vi "Functional Test Aging.vi"(8 "connection information":path, 9 "error in":errorcluster, 10 "Arduino":refnum<visa-resource-name>, 11 "System Number":string) -> (1 "error out":errorcluster, 2 "Arduino":refnum<visa-resource-name>, 3 "Functional Test Data":string)   [LabVIEW 2024]
uses:
  <vilib>/addons/database/Connection.llb/DB Tools Open Connec (Path).vi
  <vilib>/addons/database/_DB Variant To Data/Database Variant To Data.xnode
  <vilib>/addons/database/NI_Database_API.lvlib
panel:
  out "Functional Test Data Rack 1":string
  out "Functional Test Data Rack 2":string
  out "Upper Position":i32
  out "Upper Rack":dbl
  out "Lower Rack":dbl
  out "Lower Position":i32
  out "OscVoltage":string
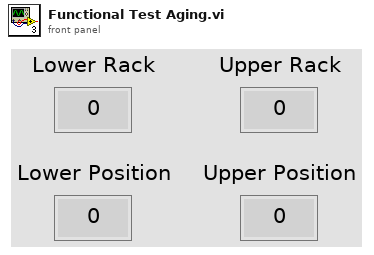
[diagram p1: front panel]
types:
  T1 = typedef "NI_Database_API.lvlib/Conn ObjectReference.ctl" = refnum<k1>
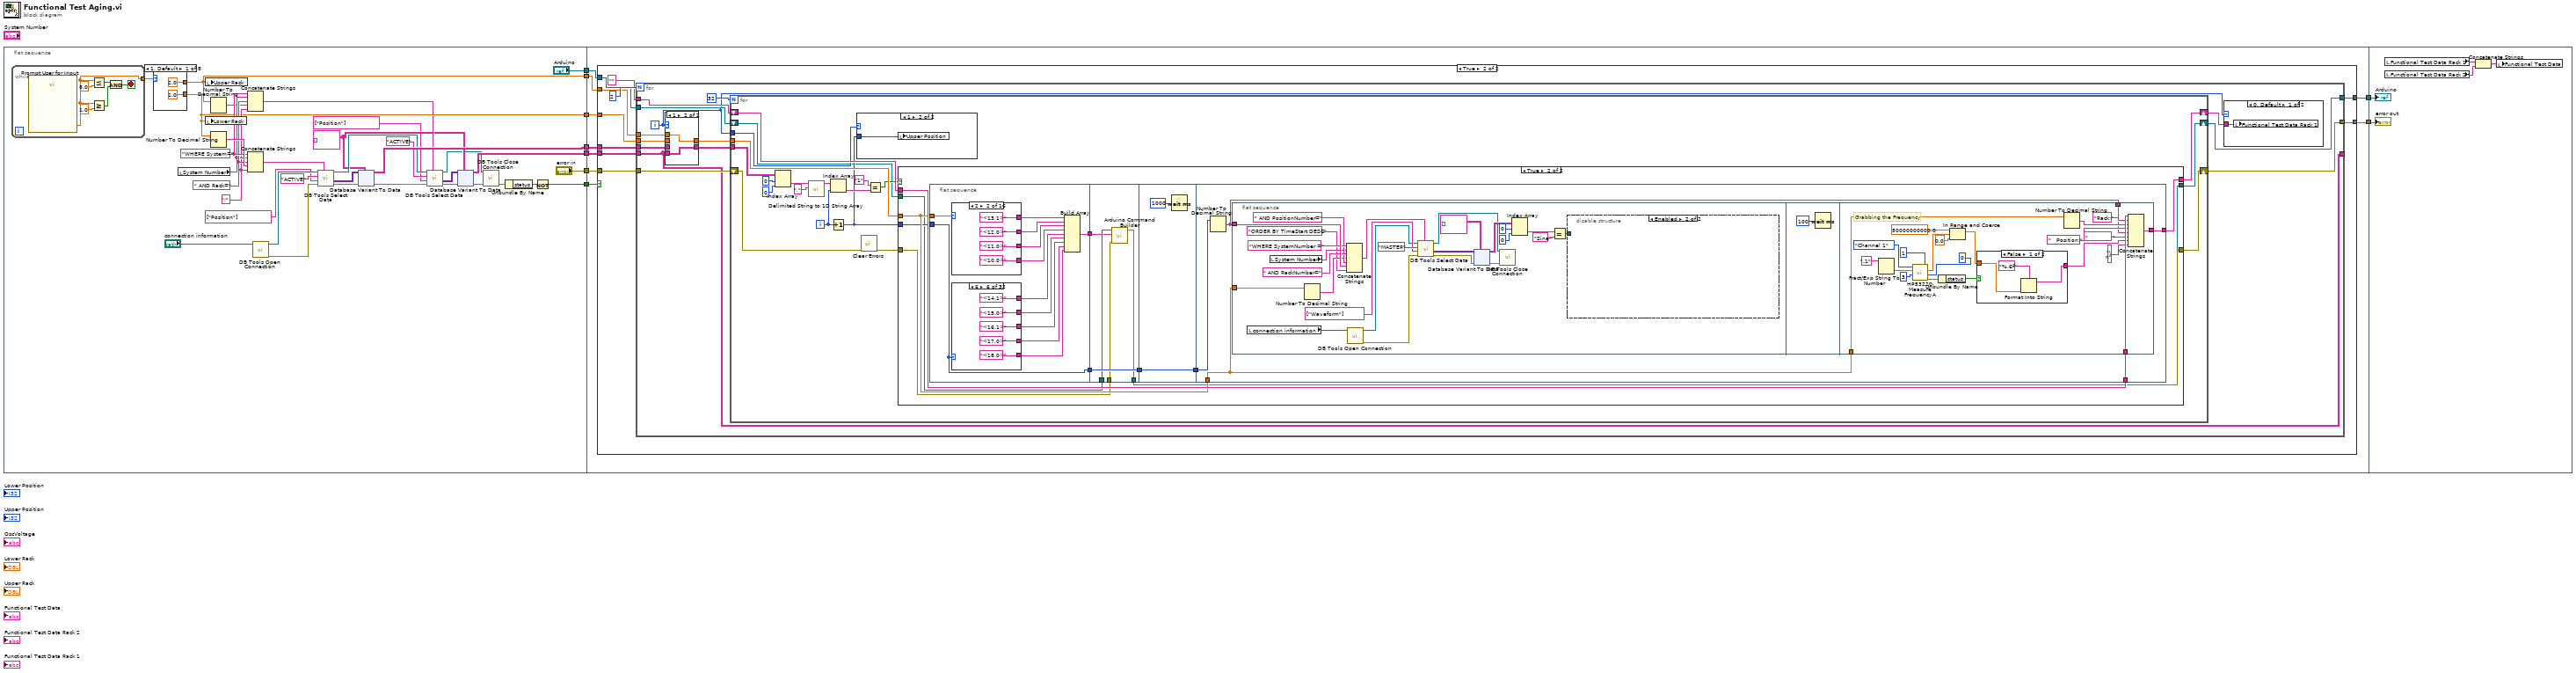
[diagram p0: block diagram]
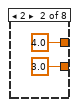
[diagram p2: hidden frame]
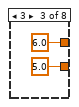
[diagram p3: hidden frame]
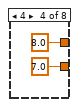
[diagram p4: hidden frame]
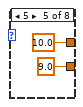
[diagram p5: hidden frame]
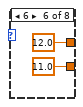
[diagram p6: hidden frame]
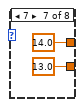
[diagram p7: hidden frame]
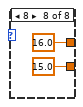
[diagram p8: hidden frame]
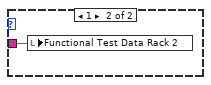
[diagram p10: hidden frame]
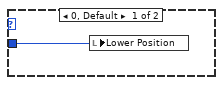
[diagram p12: hidden frame]
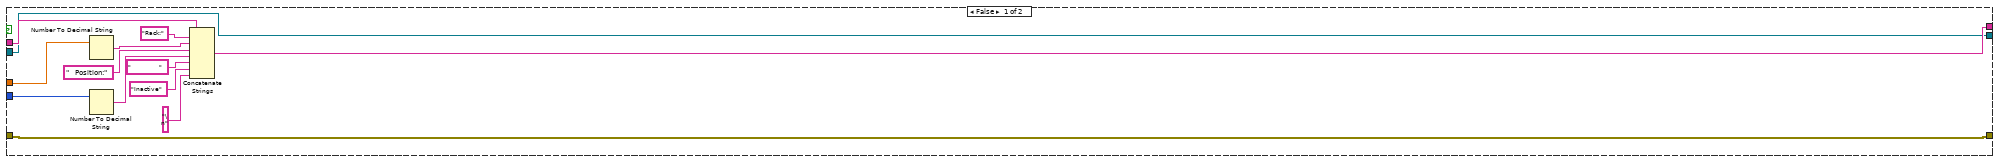
[diagram p13: hidden frame]
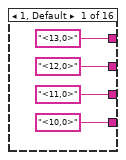
[diagram p14: hidden frame]
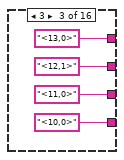
[diagram p15: hidden frame]
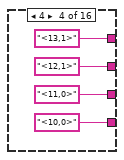
[diagram p16: hidden frame]
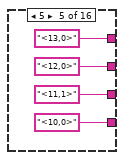
[diagram p17: hidden frame]
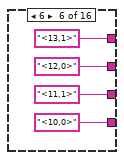
[diagram p18: hidden frame]
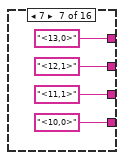
[diagram p19: hidden frame]
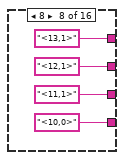
[diagram p20: hidden frame]
diagram:
  n1 = flat-sequence {
    tunnel: [w24] -> w9
    tunnel: ["Arduino"] -> w8
    tunnel: ["error in"] -> w7
    tunnel: [w16] -> w6
    tunnel: [w33] -> w5
    tunnel: [w35] -> w4
    tunnel: [w31] -> w1
    tunnel: w9 -> [w160]
    tunnel: w8 -> [w156]
    tunnel: w7 -> [w155]
    tunnel: w6 -> [w159]
    tunnel: w5 -> [w158]
    tunnel: w4 -> [w157]
    tunnel: [w162] -> w3
    tunnel: [w161] -> w2
    tunnel: w1 -> [w154]
    tunnel: w3 -> [w603]
    tunnel: w2 -> [w604]
    frame #0 {
      w15 = string[][] [] ("table")
      w39 = " AND Rack="
      w37 = ";" ("string")
      w40 = "WHERE System=" ("SQL Query")
      n2 = while {
        tunnel: [w153] -> w36
        stop <- w150 stop-if-true
        n3 = call "Prompt User for Input"() -> ("Shelf Number"=w153:dbl)  [unwired: 17 in, 2 out]
        n4 = Less Or Equal?(x=w153, y=8.0) -> (x <= y?=w149:bool)
        n5 = Greater Or Equal?(x=w153, y=1.0) -> (x >= y?=w148:bool)
        n6 = And(x=w149, y=w148) -> (x .and. y?=w150:bool)
      }
      n7 = case shown="1, Default" w36 {
        tunnel: [1.0 ("y") 3.0 ("y") 5.0 ("y") 7.0 ("y") 9.0 ("y") 11.0 ("y") 13.0 ("y") 15.0 ("y")] -> w35
        tunnel: [2.0 ("y") 4.0 ("y") 6.0 ("y") 8.0 ("y") 10.0 ("y") 12.0 ("y") 14.0 ("y") 16.0 ("y")] -> w33
        frame 1, Default {
        }
        frame 2 {
        }
        frame 3 {
        }
        frame 4 {
        }
        frame 5 {
        }
        frame 6 {
        }
        frame 7 {
        }
        frame 8 {
        }
      }
      n8 = local read "System Number"() -> (w38:string)
      n9 = local write "Upper Rack"(w33) -> ()
      n10 = local write "Lower Rack"(w35) -> ()
      n11 = Number To Decimal String(number=w33) -> (decimal integer string=w34:string)  [unwired: 1 in]
      n12 = Number To Decimal String(number=w35) -> (decimal integer string=w43:string)  [unwired: 1 in]
      n13 = Concatenate Strings(w40, w38, w39, w34, w37) -> (w21:string)
      n14 = Concatenate Strings(w40, w38, w39, w43, w37) -> (w25:string)
      n15 = call-poly <vilib>:"DB Tools Open Connection.vi"("connection information"="connection information") -> ("error out"=w28:errorcluster, "connection reference"=w29:T1)  [unwired: 7 in]
      n16 = call <vilib>:"DB Tools Select Data.vi"("condition"=w25, "error in (no error)"=w28, "columns"=string[] ["Position"], "table"="ACTIVE", "connection reference"=w29) -> ("error out"=w20:errorcluster, "data"=w26:variant[][], "connection reference out"=w23:T1)  [unwired: 1 in]
      n17 = xnode "Database Variant To Data"("database variant"=w26, "error in (no error)"=w20, "type"=w15) -> ("data"=w24:string[][], "error out"=w19:errorcluster)
      n18 = call <vilib>:"DB Tools Select Data.vi"("condition"=w21, "error in (no error)"=w19, "columns"=string[] ["Position"], "table"="ACTIVE", "connection reference"=w23) -> ("error out"=w18:errorcluster, "data"=w17:variant[][], "connection reference out"=w12:T1)  [unwired: 1 in]
      n19 = xnode "Database Variant To Data"("database variant"=w17, "error in (no error)"=w18, "type"=w15) -> ("data"=w16:string[][], "error out"=w11:errorcluster)
      n20 = call <vilib>:"DB Tools Close Connection.vi"("error in (no error)"=w11, "connection reference"=w12) -> ("error out"=w10:errorcluster)  [unwired: 5 in]
      n21 = Unbundle By Name(w10) -> ("status"=w32:bool)
      n22 = Not(x=w32) -> (.not. x?=w31:bool)
    }
    frame #1 {
      n23 = case shown="True" w154 {
        tunnel: [w163 w172] -> w162
        tunnel: [w164 w171] -> w161
        tunnel: w160 -> [_ w170]
        tunnel: w159 -> [_ w169]
        tunnel: w158 -> [_ w168]
        tunnel: w157 -> [_ w167]
        tunnel: w156 -> [w163 w166]
        tunnel: w155 -> [w164 w165]
        frame False {
        }
        frame True {
          n24 = for {
            N: 2 -> [_]
            tunnel: "" -> [w188]
            tunnel: [w187] -> w172
            tunnel: [w186] -> w171
            tunnel: w170 -> [w182]
            tunnel: w165 -> [w184]
            tunnel: w166 -> [w183]
            tunnel: [w177] -> _
            tunnel: w169 -> [w177]
            tunnel: w168 -> [w176]
            tunnel: w167 -> [w175]
            i -> [w178]
            n25 = case shown="1" w178 {
              tunnel: w182 -> [w192 _]
              tunnel: w177 -> [_ w194]
              tunnel: [w192 w194] -> w181
              tunnel: w176 -> [_ w193]
              tunnel: w175 -> [w191 _]
              tunnel: [w191 w193] -> w180
              frame 0, Default {
              }
              frame 1 {
              }
            }
            n26 = for {
              N: 32 -> [_]
              shift-right: [w203] -> w179
              shift-left: w188 -> [w204]
              tunnel: w180 -> [w205]
              tunnel: w181 -> [w209]
              shift-right: [w201] -> w187
              shift-left: w183 -> [w196]
              shift-right: [w202] -> w186
              shift-left: w184 -> [w214]
              tunnel: w178 -> [w197]
              i -> [w199]
              n27 = Index Array(array=w209, index (row)=0 ("disabled index (row)"), index (col)=0 ("disabled index (col)")) -> (element=w211:string)
              n28 = call <vilib>:"Delimited String to 1D String Array.vi"("delimiter"=",", "delimited string"=w211) -> ("string array"=w212:string[])  [unwired: 9 in]
              n29 = Index Array(array=w212, index=w199) -> (element=w213:string)
              n30 = Increment(x=w199) -> (x+1=w198:i32)
              n31 = case shown="1" w197 {
                tunnel: w198 -> [w215 w216]
                frame 0, Default {
                  n32 = local write "Lower Position"(w215) -> ()
                }
                frame 1 {
                  n33 = local write "Upper Position"(w216) -> ()
                }
              }
              n34 = call <vilib>:"Clear Errors.vi"("error in (no error)"=w214) -> ("error out"=w195:errorcluster)  [unwired: 5 in, 1 out]
              n35 = Equal?(x="1", y=w213) -> (x = y?=w200:bool)
              n36 = case shown="True" w200 {
                tunnel: w198 -> [w217 w238]
                tunnel: w205 -> [w220 w240]
                tunnel: w204 -> [w221 w241]
                tunnel: w196 -> [w218 w235]
                tunnel: w195 -> [w219 w236]
                tunnel: [w223 w239] -> w203
                tunnel: [w219 w234] -> w202
                tunnel: [w218 w233] -> w201
                frame False {
                  n37 = Number To Decimal String(number=w220) -> (decimal integer string=w228:string)  [unwired: 1 in]
                  n38 = Number To Decimal String(number=w217) -> (decimal integer string=w222:string)  [unwired: 1 in]
                  n39 = Concatenate Strings(w221, "Rack:" ("string"), w228, "   Position:" ("string"), w222, "              " ("string"), "Inactive" ("string"), "\n" ("string")) -> (w223:string)
                }
                frame True {
                  n40 = flat-sequence {
                    tunnel: w238 -> [w243]
                    tunnel: w240 -> [w244]
                    tunnel: [w243] -> w237
                    tunnel: [w242] -> w232
                    tunnel: [w483] -> w231
                    tunnel: w237 -> [w483]
                    tunnel: w236 -> [w482]
                    tunnel: w235 -> [w481]
                    tunnel: [w480] -> w234
                    tunnel: [w479] -> w233
                    tunnel: w232 -> [w478]
                    tunnel: w231 -> [w485]
                    tunnel: [w485] -> w230
                    tunnel: w241 -> [w490]
                    tunnel: w240 -> [w489]
                    tunnel: [w488] -> w239
                    tunnel: w230 -> [w486]
                    frame #0 {
                      n41 = case shown="2" w244 {
                        tunnel: ["<10,0>" ("string") "<10,0>" ("string") "<10,0>" ("string") "<10,0>" ("string") "<10,0>" ("string") "<10,0>" ("string") "<10,0>" ("string") "<10,0>" ("string") "<10,1>" ("string") "<10,1>" ("string") "<10,1>" ("string") "<10,1>" ("string") "<10,1>" ("string") "<10,1>" ("string") "<10,1>" ("string") "<10,1>" ("string")] -> w251
                        tunnel: ["<12,0>" ("string") "<12,0>" ("string") "<12,1>" ("string") "<12,1>" ("string") "<12,0>" ("string") "<12,0>" ("string") "<12,1>" ("string") "<12,1>" ("string") "<12,0>" ("string") "<12,0>" ("string") "<12,1>" ("string") "<12,1>" ("string") "<12,0>" ("string") "<12,0>" ("string") "<12,1>" ("string") "<12,1>" ("string")] -> w252
                        tunnel: ["<11,0>" ("string") "<11,0>" ("string") "<11,0>" ("string") "<11,0>" ("string") "<11,1>" ("string") "<11,1>" ("string") "<11,1>" ("string") "<11,1>" ("string") "<11,0>" ("string") "<11,0>" ("string") "<11,0>" ("string") "<11,0>" ("string") "<11,1>" ("string") "<11,1>" ("string") "<11,1>" ("string") "<11,1>" ("string")] -> w253
                        tunnel: ["<13,0>" ("string") "<13,1>" ("string") "<13,0>" ("string") "<13,1>" ("string") "<13,0>" ("string") "<13,1>" ("string") "<13,0>" ("string") "<13,1>" ("string") "<13,0>" ("string") "<13,1>" ("string") "<13,0>" ("string") "<13,1>" ("string") "<13,0>" ("string") "<13,1>" ("string") "<13,0>" ("string") "<13,1>" ("string")] -> w250
                        frame 1, Default {
                        }
                        frame 2 {
                        }
                        frame 3 {
                        }
                        frame 4 {
                        }
                        frame 5 {
                        }
                        frame 6 {
                        }
                        frame 7 {
                        }
                        frame 8 {
                        }
                        frame 9 {
                        }
                        frame 10 {
                        }
                        frame 11 {
                        }
                        frame 12 {
                        }
                        frame 13 {
                        }
                        frame 14 {
                        }
                        frame 15 {
                        }
                        frame 16 {
                        }
                      }
                      n42 = case shown="6" w243 {
                        tunnel: ["<14,0>" ("string") "<14,1>" ("string") "<14,0>" ("string") "<14,1>" ("string") "<14,0>" ("string") "<14,1>" ("string") "<14,0>" ("string") "<14,1>" ("string") "<14,0>" ("string") "<14,1>" ("string") "<14,0>" ("string") "<14,1>" ("string") "<14,0>" ("string") "<14,1>" ("string") "<14,0>" ("string") "<14,1>" ("string") "<14,0>" ("string") "<14,1>" ("string") "<14,0>" ("string") "<14,1>" ("string") "<14,0>" ("string") "<14,1>" ("string") "<14,0>" ("string") "<14,1>" ("string") "<14,0>" ("string") "<14,1>" ("string") "<14,0>" ("string") "<14,1>" ("string") "<14,0>" ("string") "<14,1>" ("string") "<14,0>" ("string") "<14,1>" ("string")] -> w249
                        tunnel: ["<16,0>" ("string") "<16,0>" ("string") "<16,0>" ("string") "<16,0>" ("string") "<16,1>" ("string") "<16,1>" ("string") "<16,1>" ("string") "<16,1>" ("string") "<16,0>" ("string") "<16,0>" ("string") "<16,0>" ("string") "<16,0>" ("string") "<16,1>" ("string") "<16,1>" ("string") "<16,1>" ("string") "<16,1>" ("string") "<16,0>" ("string") "<16,0>" ("string") "<16,0>" ("string") "<16,0>" ("string") "<16,1>" ("string") "<16,1>" ("string") "<16,1>" ("string") "<16,1>" ("string") "<16,0>" ("string") "<16,0>" ("string") "<16,0>" ("string") "<16,0>" ("string") "<16,1>" ("string") "<16,1>" ("string") "<16,1>" ("string") "<16,1>" ("string")] -> w247
                        tunnel: ["<18,0>" ("string") "<18,0>" ("string") "<18,0>" ("string") "<18,0>" ("string") "<18,0>" ("string") "<18,0>" ("string") "<18,0>" ("string") "<18,0>" ("string") "<18,0>" ("string") "<18,0>" ("string") "<18,0>" ("string") "<18,0>" ("string") "<18,0>" ("string") "<18,0>" ("string") "<18,0>" ("string") "<18,0>" ("string") "<18,1>" ("string") "<18,1>" ("string") "<18,1>" ("string") "<18,1>" ("string") "<18,1>" ("string") "<18,1>" ("string") "<18,1>" ("string") "<18,1>" ("string") "<18,1>" ("string") "<18,1>" ("string") "<18,1>" ("string") "<18,1>" ("string") "<18,1>" ("string") "<18,1>" ("string") "<18,1>" ("string") "<18,1>" ("string")] -> w245
                        tunnel: ["<15,0>" ("string") "<15,0>" ("string") "<15,1>" ("string") "<15,1>" ("string") "<15,0>" ("string") "<15,0>" ("string") "<15,1>" ("string") "<15,1>" ("string") "<15,0>" ("string") "<15,0>" ("string") "<15,1>" ("string") "<15,1>" ("string") "<15,0>" ("string") "<15,0>" ("string") "<15,1>" ("string") "<15,1>" ("string") "<15,0>" ("string") "<15,0>" ("string") "<15,1>" ("string") "<15,1>" ("string") "<15,0>" ("string") "<15,0>" ("string") "<15,1>" ("string") "<15,1>" ("string") "<15,0>" ("string") "<15,0>" ("string") "<15,1>" ("string") "<15,1>" ("string") "<15,0>" ("string") "<15,0>" ("string") "<15,1>" ("string") "<15,1>" ("string")] -> w248
                        tunnel: ["<17,0>" ("string") "<17,0>" ("string") "<17,0>" ("string") "<17,0>" ("string") "<17,0>" ("string") "<17,0>" ("string") "<17,0>" ("string") "<17,0>" ("string") "<17,1>" ("string") "<17,1>" ("string") "<17,1>" ("string") "<17,1>" ("string") "<17,1>" ("string") "<17,1>" ("string") "<17,1>" ("string") "<17,1>" ("string") "<17,0>" ("string") "<17,0>" ("string") "<17,0>" ("string") "<17,0>" ("string") "<17,0>" ("string") "<17,0>" ("string") "<17,0>" ("string") "<17,0>" ("string") "<17,1>" ("string") "<17,1>" ("string") "<17,1>" ("string") "<17,1>" ("string") "<17,1>" ("string") "<17,1>" ("string") "<17,1>" ("string") "<17,1>" ("string")] -> w246
                        frame 1, Default {
                        }
                        frame 2 {
                        }
                        frame 3 {
                        }
                        frame 4 {
                        }
                        frame 5 {
                        }
                        frame 6 {
                        }
                        frame 7 {
                        }
                        frame 8 {
                        }
                        frame 9 {
                        }
                        frame 10 {
                        }
                        frame 11 {
                        }
                        frame 12 {
                        }
                        frame 13 {
                        }
                        frame 14 {
                        }
                        frame 15 {
                        }
                        frame 16 {
                        }
                        frame 17 {
                        }
                        frame 18 {
                        }
                        frame 19 {
                        }
                        frame 20 {
                        }
                        frame 21 {
                        }
                        frame 22 {
                        }
                        frame 23 {
                        }
                        frame 24 {
                        }
                        frame 25 {
                        }
                        frame 26 {
                        }
                        frame 27 {
                        }
                        frame 28 {
                        }
                        frame 29 {
                        }
                        frame 30 {
                        }
                        frame 31 {
                        }
                        frame 32 {
                        }
                      }
                      n43 = Build Array(w250, w252, w253, w251, w249, w248, w247, w246, w245) -> (w242:string[])
                    }
                    frame #1 {
                      n44 = call "Arduino Command Builder.vi"("error in"=w482, "Commands"=w478, "Arduino in"=w481) -> ("error out"=w480:errorcluster, "Arduino out"=w479:refnum<visa-resource-name>)  [unwired: 7 in]
                    }
                    frame #2 {
                      n45 = Wait (ms)(milliseconds to wait=u32 1000) -> ()  [unwired: 1 out]
                    }
                    frame #3 {
                      n46 = Number To Decimal String(number=w486) -> (decimal integer string=w487:string)  [unwired: 1 in]
                      n47 = flat-sequence {
                        tunnel: w489 -> [w515]
                        tunnel: w487 -> [w514]
                        tunnel: [w595] -> w488
                        tunnel: w489 -> [w576]
                        tunnel: w490 -> [w593]
                        tunnel: w487 -> [w577]
                        frame #0 {
                          n48 = local read "connection information"() -> (w491:path)
                          n49 = local read "System Number"() -> (w509:string)
                          n50 = Number To Decimal String(number=w515) -> (decimal integer string=w508:string)  [unwired: 1 in]
                          n51 = Concatenate Strings("WHERE SystemNumber =" ("SQL Query"), w509, " AND RackNumber=" ("string"), w508, " AND PositionNumber=" ("string"), w514, "ORDER BY TimeStart DESC" ("string")) -> (w499:string)
                          n52 = call-poly <vilib>:"DB Tools Open Connection.vi"("connection information"=w491) -> ("error out"=w494:errorcluster, "connection reference"=w495:T1)  [unwired: 7 in]
                          n53 = call <vilib>:"DB Tools Select Data.vi"("condition"=w499, "error in (no error)"=w494, "columns"=string[] ["Waveform"], "table"="MASTER", "connection reference"=w495) -> ("error out"=w500:errorcluster, "data"=w501:variant[][], "connection reference out"=w493:T1)  [unwired: 1 in]
                          n54 = xnode "Database Variant To Data"("database variant"=w501, "error in (no error)"=w500, "type"=string[][] [] ("table")) -> ("data"=w498:string[][], "error out"=w492:errorcluster)
                          n55 = call <vilib>:"DB Tools Close Connection.vi"("error in (no error)"=w492, "connection reference"=w493) -> ()  [unwired: 5 in, 1 out]
                          n56 = Index Array(array=w498, index (row)=0, index (col)=0) -> (element=w504:string)
                          n57 = Equal?(x=w504, y="Sine") -> (x = y?=w513:bool)
                          n58 = disable-structure shown="Enabled" {
                            disable-tunnel: w513 -> [w516 _]
                            frame Disabled {
                              n59 = case shown="False" w516 {
                                frame False {
                                n60 = flat-sequence {
                                frame #0 {
                                n61 = Send(0:0 ("bus"), 2:i16 3 ("address"), 5:"INP1:COUP DC " ("data string")) -> ()  [unwired: 2 in, 3 out]
                                }
                                frame #1 {
                                n62 = Send(0:0 ("bus"), 2:i16 3 ("address"), 5:"INP1:IMP MAX" ("data string")) -> ()  [unwired: 2 in, 3 out]
                                }
                                }
                                }
                                frame True {
                                n63 = flat-sequence {
                                frame #0 {
                                n64 = Send(0:0 ("bus"), 2:i16 3 ("address"), 5:"INP1:COUP AC " ("data string")) -> ()  [unwired: 2 in, 3 out]
                                }
                                frame #1 {
                                n65 = Send(0:0 ("bus"), 2:i16 3 ("address"), 5:"INP1:IMP MIN" ("data string")) -> ()  [unwired: 2 in, 3 out]
                                }
                                }
                                }
                              }
                            }
                            frame Enabled {
                            }
                          }
                        }
                        frame #1 {
                          n66 = Wait (ms)(milliseconds to wait=u32 100) -> ()  [unwired: 1 out]
                        }
                        frame #2 {
                          # "Grabbing the Frequency"
                          n67 = Fract/Exp String To Number(string=".1") -> (number=w585:dbl)  [unwired: 3 in, 1 out]
                          n68 = call "HP53220 Measure FrequencyA.vi"("GPIB Bus"=0, "Number of Readings"=1, "GPIB Address"=i16 3, "Gate Time"=w585, "Channel(1,2,3)"=enum16{"Channel 1", "Channel 2", "Channel 3"}."Channel 1") -> ("error out"=w581:errorcluster, "Frequency"=w574:dbl)  [unwired: 1 in]
                          n69 = Unbundle By Name(w581) -> ("status"=w582:bool)
                          n70 = In Range and Coerce(upper limit=50000000000.0 ("y"), x=w574, lower limit=0.0) -> (coerced(x)=w575:dbl)  [unwired: 1 out]
                          n71 = case shown="False" w582 {
                            tunnel: w575 -> [w597 _]
                            tunnel: [w596 "-1"] -> w580
                            frame False {
                              n72 = Format Into String(format string="%.6f", w597) -> (resulting string=w596:string)  [unwired: 2 in, 1 out]
                            }
                            frame True {
                            }
                          }
                          n73 = Number To Decimal String(number=w576) -> (decimal integer string=w591:string)  [unwired: 1 in]
                          n74 = Concatenate Strings(w593, "Rack:" ("string"), w591, "   Position:" ("string"), w577, "              " ("string"), w580, "\n" ("string")) -> (w595:string)
                        }
                      }
                    }
                  }
                }
              }
            }
            n75 = case shown="0, Default" w178 {
              tunnel: w179 -> [w189 w190]
              frame 0, Default {
                n76 = local write "Functional Test Data Rack 1"(w189) -> ()
              }
              frame 1 {
                n77 = local write "Functional Test Data Rack 2"(w190) -> ()
              }
            }
          }
        }
      }
    }
    frame #2 {
      n78 = local read "Functional Test Data Rack 1"() -> (w601:string)
      n79 = local read "Functional Test Data Rack 2"() -> (w602:string)
      n80 = Concatenate Strings(w601, w602) -> (w600:string)
      n81 = local write "Functional Test Data"(w600) -> ()
      "Arduino" <- w603
      "error out" <- w604
    }
  }
